vi "Run Core.vi"(8 "Error In":errorcluster, 9 "Timeout (s)":dbl, 10 "IAction In":refnum<class "IAction.lvclass">, 11 "Reference In":refnum<class "IRef.lvclass">) -> (0 "Error Out":errorcluster, 1 "Timeout?":bool, 2 "IResult Out":refnum<class "IResult.lvclass">, 3 "Reference Out":refnum<class "IRef.lvclass">)   [LabVIEW 2020, in "IAction.lvclass"]
uses:
  IAction.lvclass
  IReference/IRef.lvclass
  IResult/IResult.lvclass
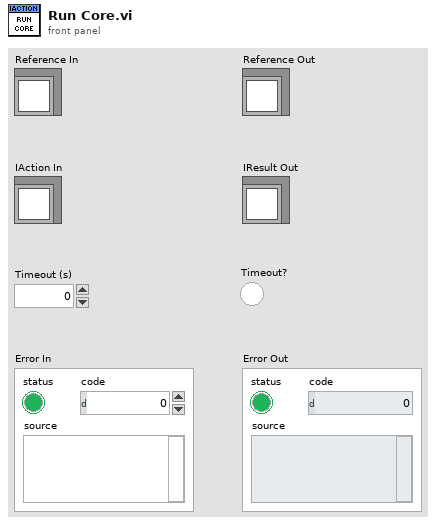
[diagram p1: front panel]
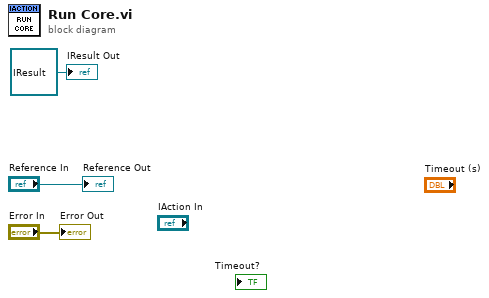
[diagram p0: block diagram]
diagram:
  "Error Out" <- "Error In"
  "Reference Out" <- "Reference In"
  "IResult Out" <- refnum<class "IResult.lvclass"> refnum ("IResult Out")
